vi "Sender IPES.vi"(8 "Relation":T1=enum."Creator", 9 "Path":path, 10 "Self Alias":string, 11 "Msg in":refnum<class "Msg.lvclass">) -> (3 "Msg out":refnum<class "Msg.lvclass">)   [LabVIEW 2021, in "jettl.lvlib" / "Msg.lvclass"]
uses:
  Msg.lvclass
  Sender/Relation.ctl
  Sender/Sender/Sender.lvclass
  Sender/Sender.lvlib
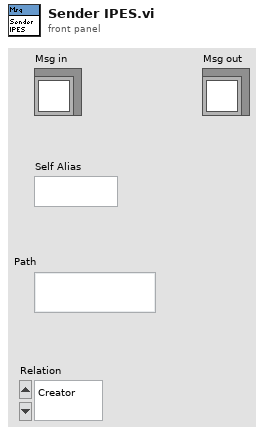
[diagram p1: front panel]
types:
  T1 = typedef "jettl.lvlib/Sender.lvlib/Relation.ctl" = enum16{"Self", "Creator", "Created"}
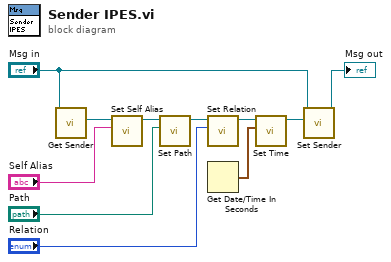
[diagram p0: block diagram]
diagram:
  n1 = call-dynamic "Get Sender.vi"("Msg in"="Msg in") -> ("Sender"=w8:refnum<class "Sender.lvclass">)  [unwired: 10 in]
  n2 = call-dynamic "Set Self Alias.vi"("Self Alias"="Self Alias", "Sender in"=w8) -> ("Sender out"=w9:refnum<class "Sender.lvclass">)  [unwired: 9 in]
  n3 = call-dynamic "Set Path.vi"("Path"="Path", "Sender in"=w9) -> ("Sender out"=w10:refnum<class "Sender.lvclass">)  [unwired: 9 in]
  n4 = call-dynamic "Set Relation.vi"("Relation"="Relation", "Sender in"=w10) -> ("Sender out"=w11:refnum<class "Sender.lvclass">)  [unwired: 9 in]
  n5 = Get Date/Time In Seconds() -> (seconds since 1Jan1904=w5:timestamp)
  n6 = call-dynamic "Set Time.vi"("Time"=w5, "Sender in"=w11) -> ("Sender out"=w7:refnum<class "Sender.lvclass">)  [unwired: 9 in]
  n7 = call-dynamic "Set Sender.vi"("Sender"=w7, "Msg in"="Msg in") -> ("Msg out"=→"Msg out":refnum<class "Msg.lvclass">)  [unwired: 9 in]
